vi "DAQmx-Lock_UnLock.vi"(8 "entrée d'erreur (pas d'erreur)":errorcluster, 10 "Control-Client old entrée":refnum<class "Control-Client.lvclass">, 11 "Control-Client new entrée":refnum<class "Control-Client.lvclass">) -> (0 "sortie d'erreur":errorcluster, 2 "Control-Client old out":refnum<class "Control-Client.lvclass">, 3 "Control-Client new out":refnum<class "Control-Client.lvclass">)   [LabVIEW 2019, in "Control-Client.lvclass"]
uses:
  Control-Client.lvclass
  Control-Client.lvclass/Control-Client.ctl
  controls/Gauge_pump/Gauge_pump.xctl
  dependecies/XControls/CellsDL/ControlDL.xctl
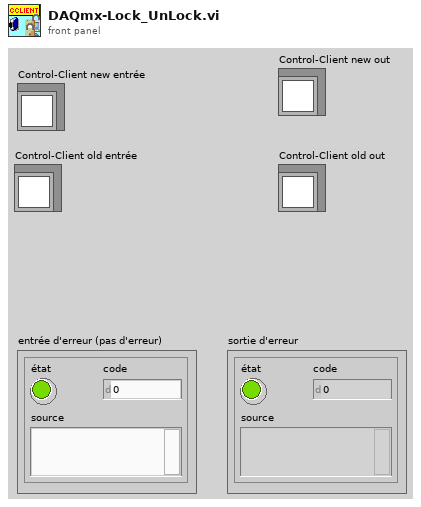
[diagram p1: front panel]
types:
  T1 = enum8{"Enabled", "Disabled", "Disabled and Grayed Out"}
  T2 = typedef "Control-Client.lvclass/Controls-with-permissions_CLIENT.ctl" = cluster{"Server ON/OFF":refnum<vi>, "Detector connect":refnum<vi>, "DL connect":refnum<vi>, "DAQmx connect":refnum<vi>, "All connect":refnum<vi>, "Start measurement":refnum<vi>, "Move Crystal":refnum<vi>, "Relay key heater":refnum<vi>, "Laser Shutter":refnum<vi>, "Accelerator Shutter":refnum<vi>, "Power":refnum<vi>, "Unlock":refnum<vi>, "RT":refnum<vi>, "Faraday Cup":refnum<vi>, "Osc connect":refnum<vi>, "ELYSE pulses":refnum<vi>, "Cells":refnum<vi>, "Pump":refnum<vi>, "# par point":refnum<vi>, "Alarm":refnum<vi>, "oscilloscopeRead":refnum<vi>, "WCM_state":refnum<vi>, "ControlDL":refnum<vi>}
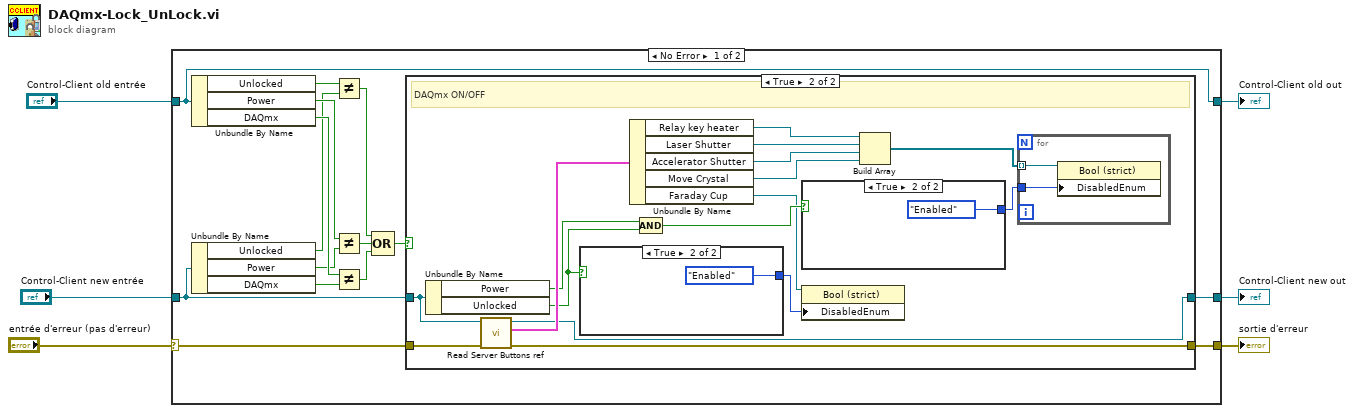
[diagram p0: block diagram]
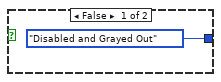
[diagram p3: hidden frame]
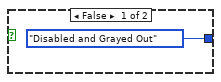
[diagram p4: hidden frame]
diagram:
  n1 = case shown="No Error" "entrée d'erreur (pas d'erreur)" {
    selector: "entrée d'erreur (pas d'erreur)" -> [w8 w48]
    tunnel: [w21 w48] -> w6
    tunnel: "Control-Client new entrée" -> [w16 w47]
    tunnel: [w9 w47] -> w4
    tunnel: "Control-Client old entrée" -> [w7 w46]
    tunnel: [w7 w46] -> w1
    frame No Error {
      n2 = Unbundle By Name(w7) -> ("Unlocked"=w11:bool, "Power"=w18:bool, "DAQmx"=w19:bool)
      n3 = Unbundle By Name(w16) -> ("Unlocked"=w10:bool, "Power"=w17:bool, "DAQmx"=w20:bool)
      n4 = Not Equal?(x=w11, y=w10) -> (x != y?=w15:bool)
      n5 = Not Equal?(x=w18, y=w17) -> (x != y?=w14:bool)
      n6 = Not Equal?(x=w19, y=w20) -> (x != y?=w13:bool)
      n7 = Compound Arithmetic op=OR ("Opérateur arithmétique")(w15, w14, w13) -> (w12:bool)
      n8 = case shown="True" w12 {
        tunnel: w16 -> [w22 w25]
        tunnel: w8 -> [w23 w32]
        tunnel: [w23 w31] -> w21
        tunnel: [w22 w24] -> w9
        frame False {
        }
        frame True {
          # "DAQmx ON/OFF"
          n9 = Unbundle By Name(w25) -> ("Power"=w29:bool, "Unlocked"=w28:bool)
          n10 = call "Read Server Buttons ref.vi"("error in (no error)"=w32, "Control-Client in"=w25) -> ("error out"=w31:errorcluster, "Server Buttons ref"=w39:T2, "Control-Client out"=w24:refnum<class "Control-Client.lvclass">)  [unwired: 7 in]
          n11 = case shown="True" w28 {
            tunnel: [T1."Disabled and Grayed Out" ("Désactivé") T1."Enabled" ("Désactivé")] -> w27
            frame False {
            }
            frame True {
            }
          }
          n12 = Unbundle By Name(w39) -> ("Relay key heater"=w33:refnum<vi>, "Laser Shutter"=w34:refnum<vi>, "Accelerator Shutter"=w35:refnum<vi>, "Move Crystal"=w36:refnum<vi>, "Faraday Cup"=w26:refnum<vi>)
          n13 = Compound Arithmetic op=AND(w29, w28) -> (w30:bool)
          n14 = case shown="True" w30 {
            tunnel: [T1."Disabled and Grayed Out" ("Désactivé") T1."Enabled" ("Désactivé")] -> w38
            frame False {
            }
            frame True {
            }
          }
          n15 = property class="Bool (strict)"(reference=w26, "DisabledEnum"=w27) -> ()  [unwired: 1 in, 2 out]
          n16 = Build Array(w33, w34, w35, w36) -> (w37:refnum<vi>[])
          n17 = for {
            tunnel: w37 -> [w45] mode=indexing
            tunnel: w38 -> [w44]
            n18 = property class="Bool (strict)"(reference=w45, "DisabledEnum"=w44) -> ()  [unwired: 1 in, 2 out]
          }
        }
      }
    }
    frame Error {
    }
  }
  "sortie d'erreur" <- w6
  "Control-Client new out" <- w4
  "Control-Client old out" <- w1
